vi "Sine.vi"() -> ()   [LabVIEW 2023]
doc: "This example shows how the Sine function operates with different data types. These concepts also apply to the Cosine, Tangent, Secant, Cosecant, Cotangent, Inverse Sine, Inverse Cosine, Inverse Tangent, Inverse Secant, Inverse Cosecant, Inverse Cotangent, Sine & Cosine, Sinc, Inverse Tangent (2 Input) Hyperbolic Sine, Hyperbolic Cosine, Hyperbolic Tangent, Hyperbolic Secant, Hyperbolic Cosecant, Hyperbolic Cotangent, Inverse Hyperbolic Sine, Inverse Hyperbolic Cosine, Inverse Hyperbolic Tangent, Inverse Hyperbolic Secant, Inverse Hyperbolic Cosecant, and Inverse Hyperbolic Cotangent functions."
panel:
  in  "Tab Control":T1(tab)
  out "sin(x)":dbl
  in  "numeric":dbl=3.14
  out "sin(x)":dbl[](array[numeric])
  in  "Array":dbl[](array[numeric])=[1.0, 2.0, 3.0, 4.0, 5.0, 6.0]
  out "sin(x)":cluster{"numeric":dbl, "numeric 2":dbl}
  in  "Cluster":cluster{"numeric":dbl, "numeric 2":dbl}={"numeric"=4.0, "numeric 2"=6.28}
  out "sin(x)":cluster{"numeric":dbl, "numeric 2":dbl}[](array[cluster])
  in  "Array of Cluster":cluster{"numeric":dbl, "numeric 2":dbl}[](array[cluster])=[{"numeric"=2.0, "numeric 2"=6.0}, {"numeric"=1.0, "numeric 2"=3.0}, {"numeric"=3.14, "numeric 2"=6.28}]
  # "Overview: Demonstrates how the Sine function operates with different data types.\nInstructions:\n1. Run the VI.\n2. Examine the different cases.\n3. Although this example demonstrates the Sine function, the concepts also apply to other Trigonometric Functions and Hyperbolic Functions."
  # "The sine of the numeric is computed to give sin(x), where the numeric is in radians."
  # "The sine of each element in the array is computed to give an array of sin(x), where each array element is in radians."
  # "The sine of each element in the cluster is computed to give a cluster of sin(x), where each cluster element is a numeric and in radians.  A cluster of numeric arrays would produce a cluster of numeric arrays."
  # "The sine of each element in the array is computed to give an array of clusters of sin(x), where each cluster element is a numeric and in radians."
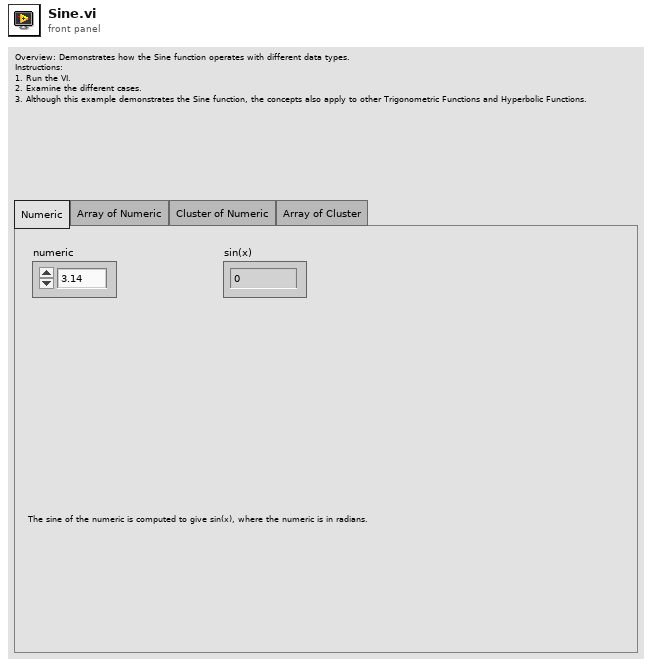
[diagram p1: front panel]
types:
  T1 = enum32{"Numeric", "Array of Numeric", "Cluster of Numeric", "Array of Cluster"}
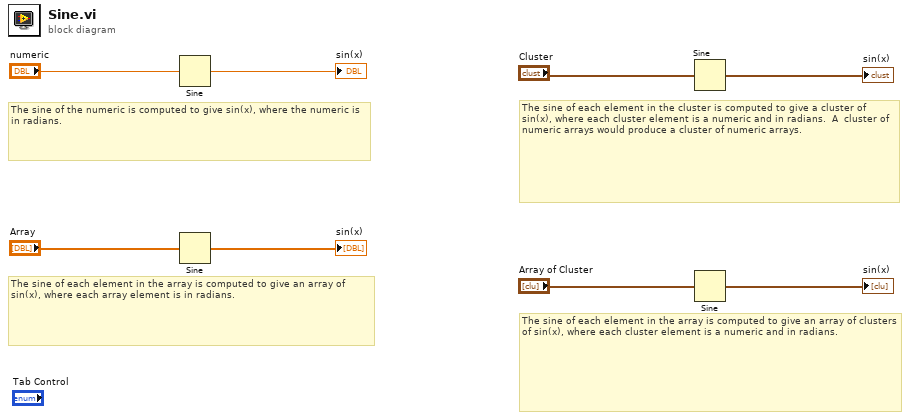
[diagram p0: block diagram]
diagram:
  # "The sine of each element in the array is computed to give an array of clusters of sin(x), where each cluster element is a numeric and in radians."
  # "The sine of each element in the cluster is computed to give a cluster of sin(x), where each cluster element is a numeric and in radians.  A  cluster of numeric arrays would produce a cluster of numeric arrays."
  # "The sine of each element in the array is computed to give an array of sin(x), where each array element is in radians."
  # "The sine of the numeric is computed to give sin(x), where the numeric is in radians."
  n1 = Sine(x="numeric") -> (sin(x)=→"sin(x)":dbl)
  n2 = Sine(x="Array") -> (sin(x)=→"sin(x)":dbl[])
  n3 = Sine(x="Cluster") -> (sin(x)=→"sin(x)":cluster{"numeric":dbl, "numeric 2":dbl})
  n4 = Sine(x="Array of Cluster") -> (sin(x)=→"sin(x)":cluster{"numeric":dbl, "numeric 2":dbl}[])
